vi "FileOpenWindow.vi"(8 "error in (no error)":errorcluster, 10 "Path In":string, 11 "Connection ID":T1) -> (0 "error out":errorcluster, 2 "Path Out":string, 3 "Connection ID Out":T1)   [LabVIEW 2017, in "GL860_Driver.lvlib"]
uses:
  GL860_Driver.lvlib
  Driver/ConnectionID.ctl
  <vilib>/Utility/miscctls.llb/LVPointTypeDef.ctl
panel:
  in  "Save File_Info":i32[](listbox) caption="Save File"
  in  "OK":bool
  in  "Scrollbar":i32(c297)
  out "Img 7":picture
  out "Img 6":picture
  out "Img 5":picture
  out "Img 4":picture
  out "Img 3":picture
  out "Img 2":picture
  out "Img 0":picture
  out "Img 1":picture
  out "Save File_Name":i32[](listbox) caption="Save File"
  in  "Tag":string
  in  "Pic.Temp":picture[](array[picture])=[bytes[7070], bytes[7070]]
  out "Icon":picture[](array[picture])
  out "DriveList":string[](array[string])
  out "File":string[](array[string])
  out "Folder":string[](array[string])
  in  "Device":i32(ring) items=["SD1"=-1, "-"=-2, "SD1"=0, "SD2"=1]
  in  "キャンセル":bool
  in  "Transfar":bool
  in  "Tree":string(tree)
  out "FilePath":string
  in  "Sort":u16(ring) items=["ファイル名", "更新日時"]
  in  "Send 3":bool
  in  "Send 4":bool
  # "ソート"
  # "デバイス"
  # "ファイルパス"
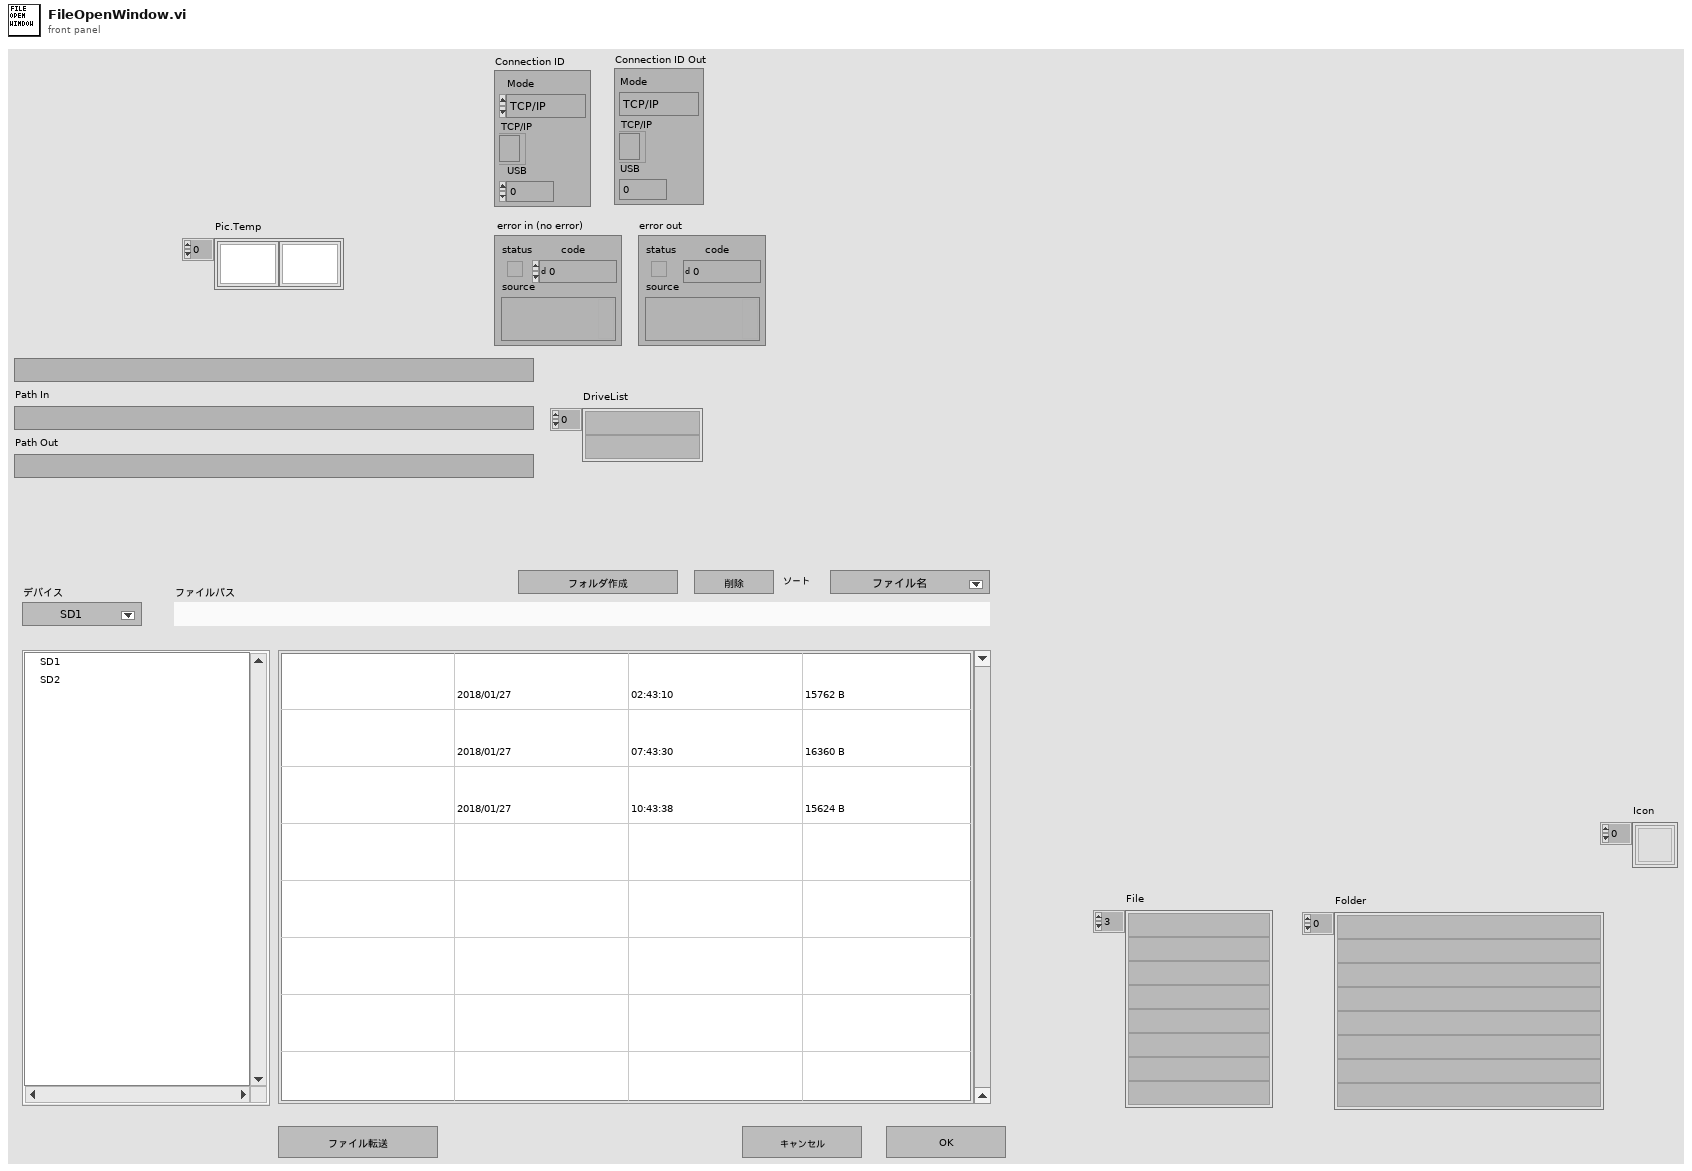
[diagram p1: front panel]
types:
  T1 = typedef "ConnectionID.ctl" = cluster{"Mode":enum16{"TCP/IP", "USB"}, "TCP/IP":refnum<k5>, "USB":i32}
  T2 = typedef "LVPointTypeDef.ctl" = cluster{"Horizontal":i16, "Vertical":i16}
  T3 = typedef "LVRowAndColumnUnsignedTypeDef.ctl" = cluster{"Row":u32, "Column":u32}
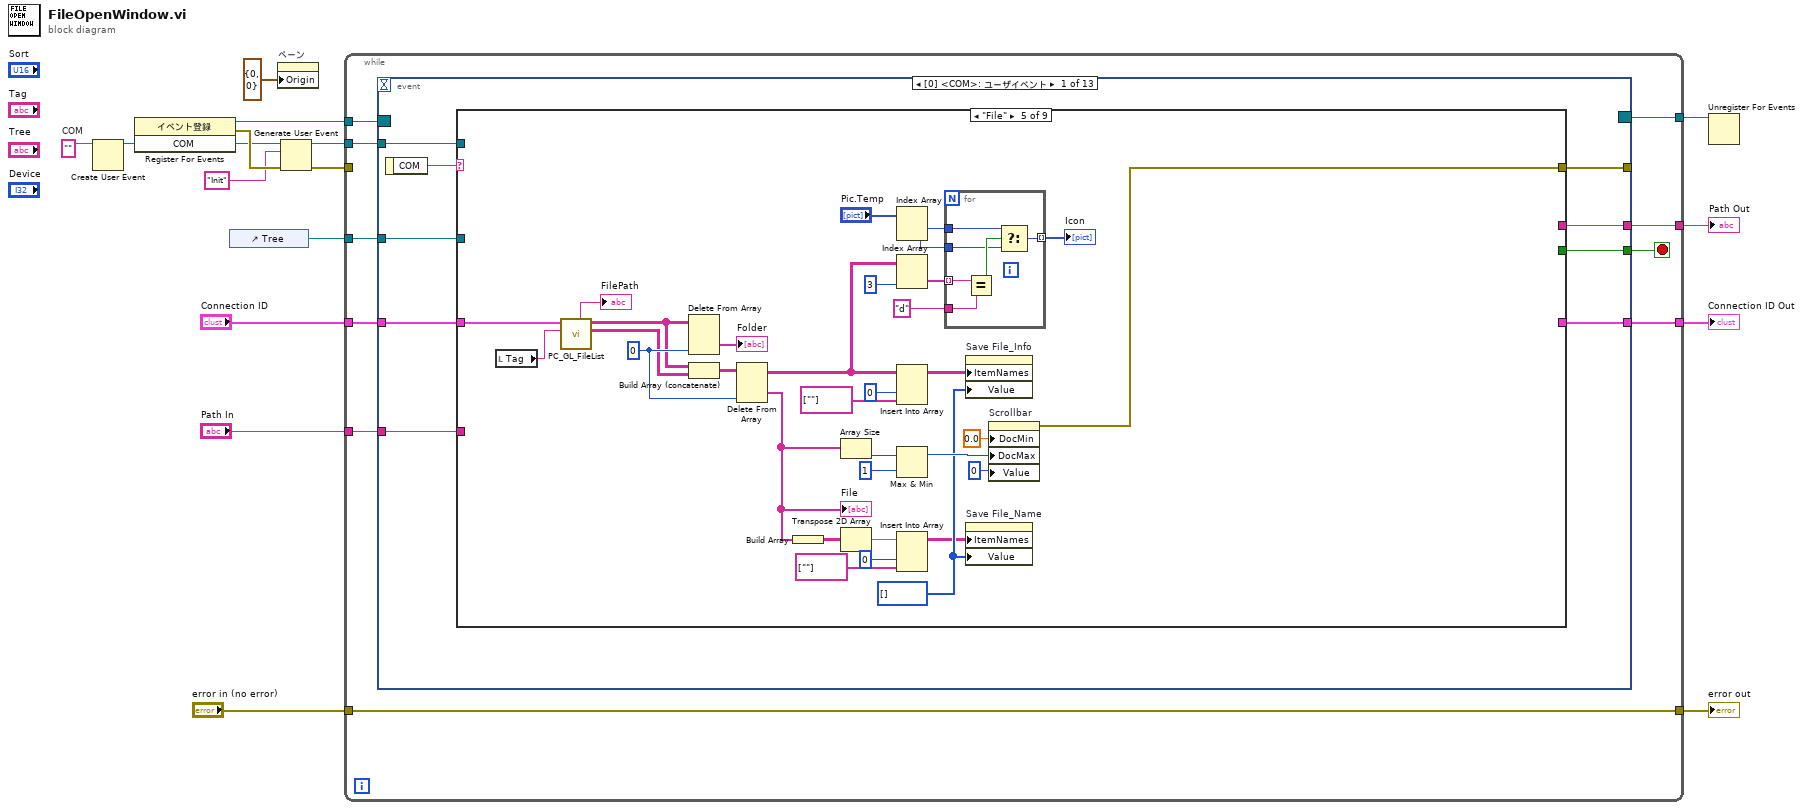
[diagram p0: block diagram]
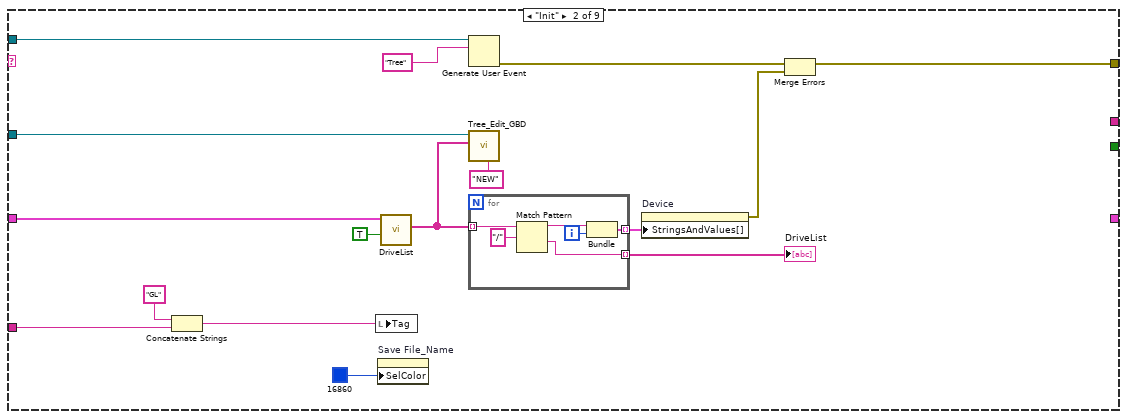
[diagram p3: hidden frame]
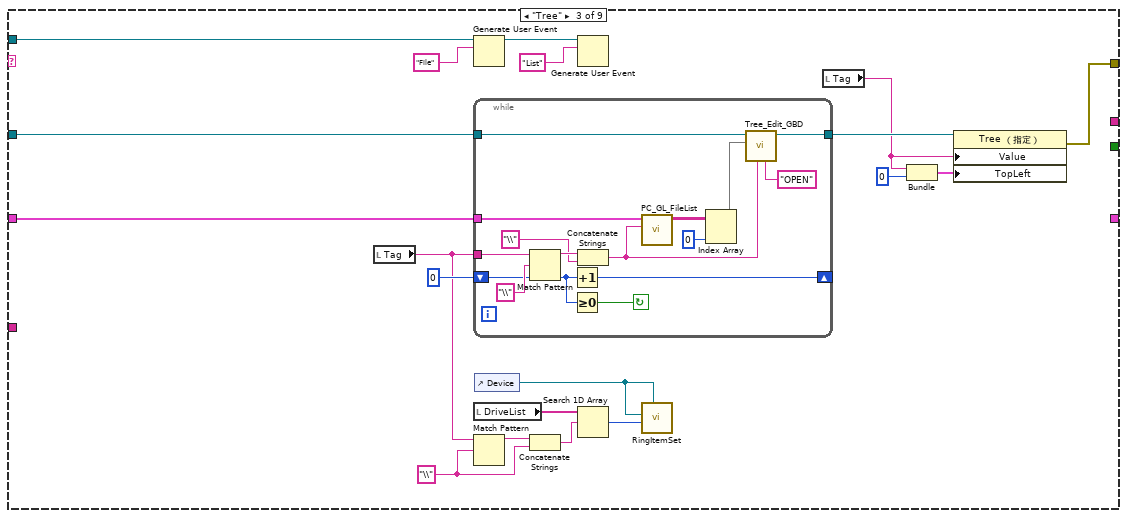
[diagram p4: hidden frame]
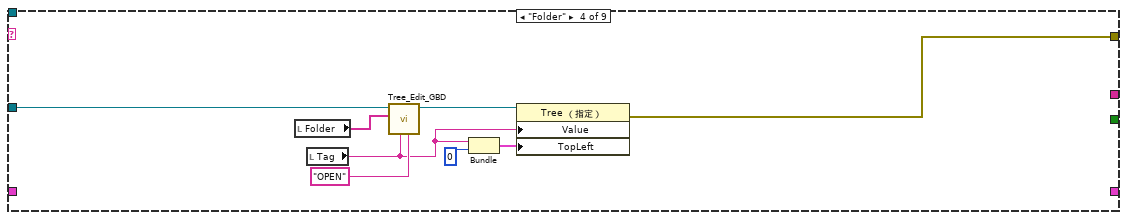
[diagram p5: hidden frame]
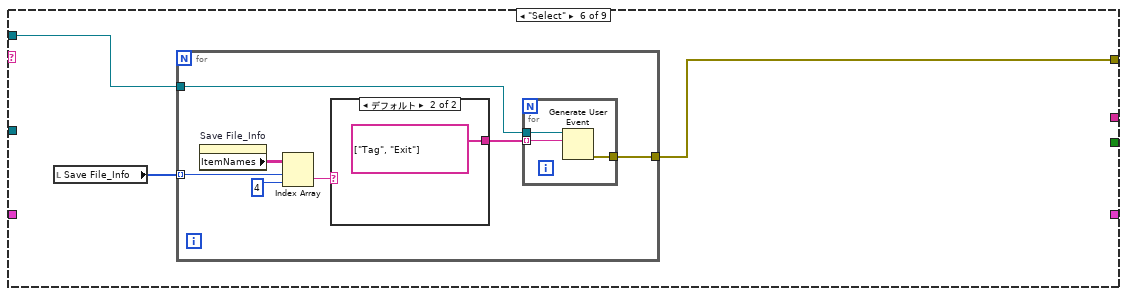
[diagram p6: hidden frame]
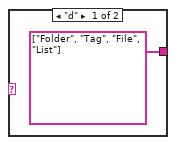
[diagram p7: hidden frame]
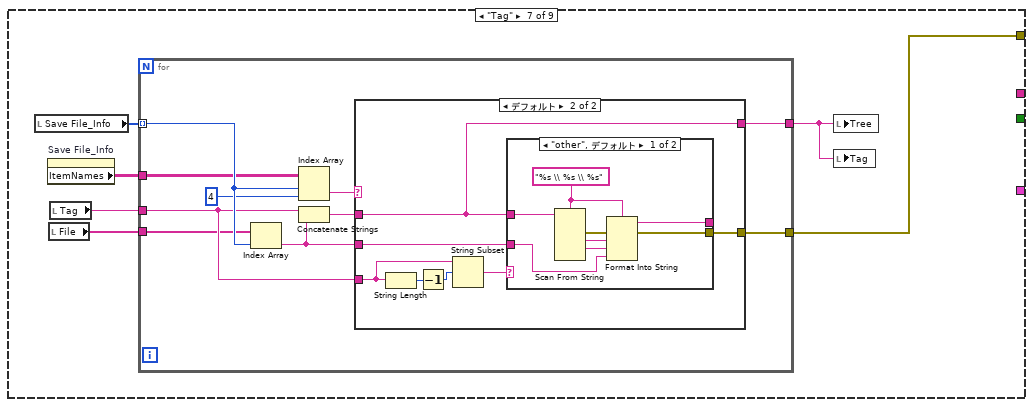
[diagram p8: hidden frame]
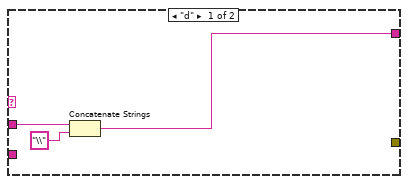
[diagram p9: hidden frame]
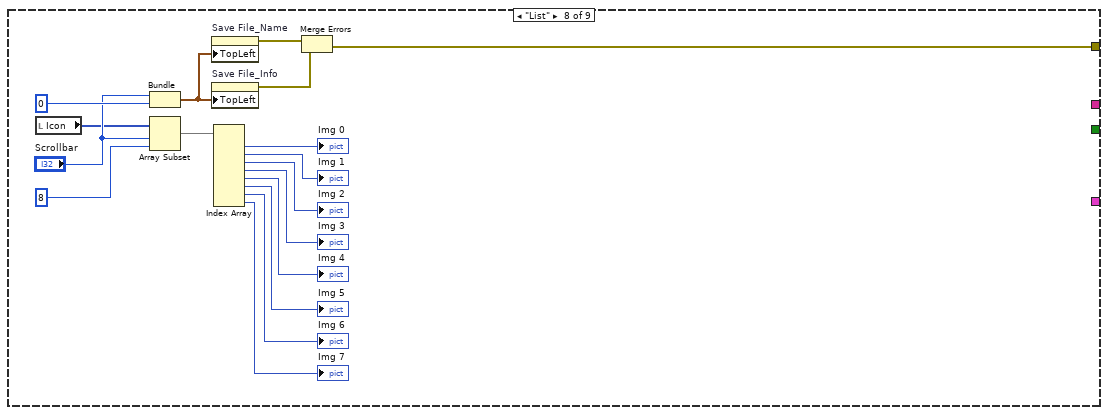
[diagram p11: hidden frame]
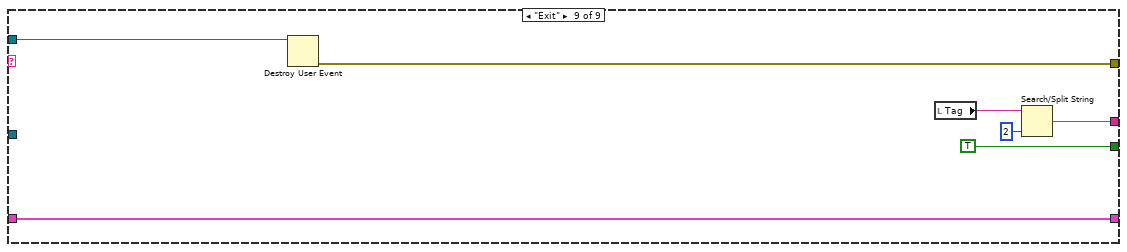
[diagram p12: hidden frame]
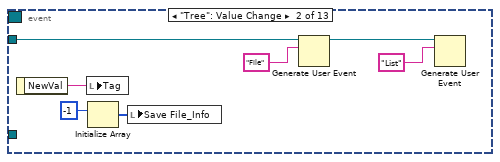
[diagram p13: hidden frame]
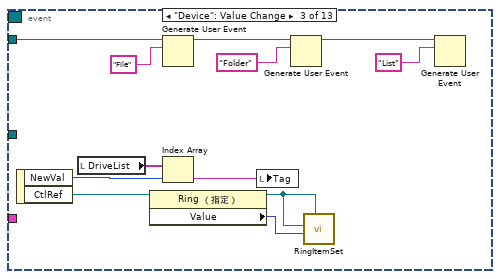
[diagram p14: hidden frame]
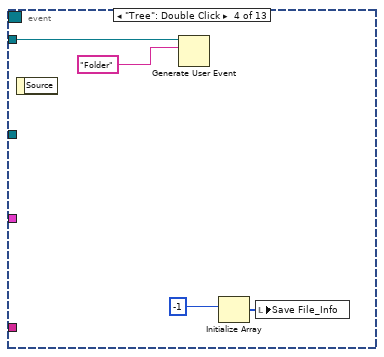
[diagram p15: hidden frame]
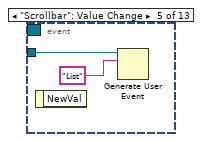
[diagram p16: hidden frame]
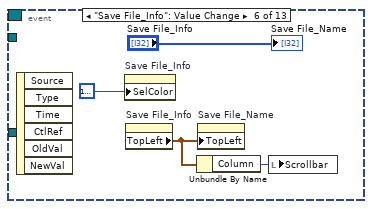
[diagram p17: hidden frame]
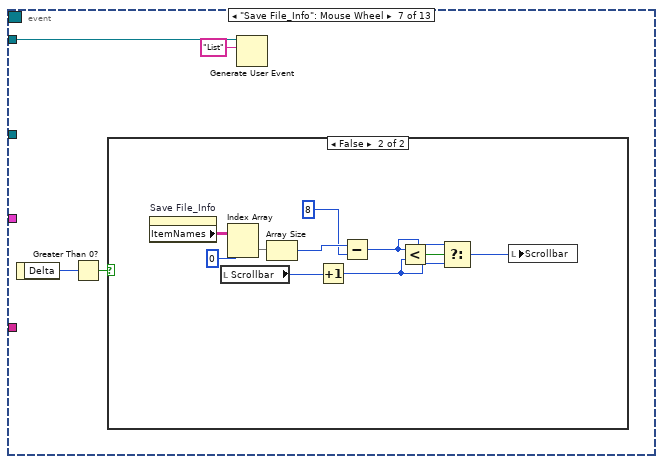
[diagram p18: hidden frame]
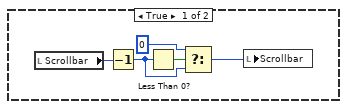
[diagram p19: hidden frame]
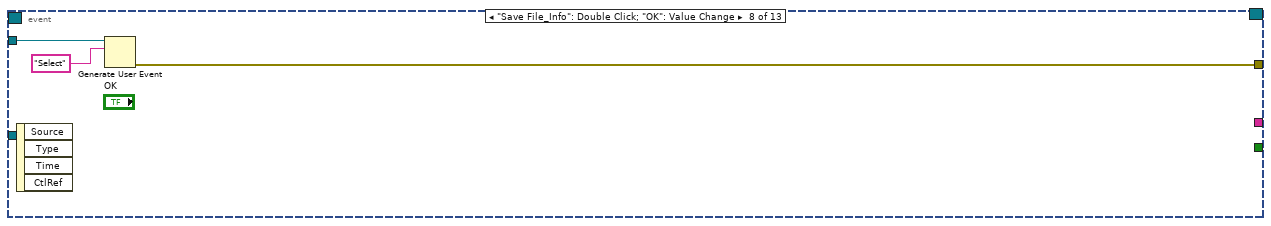
[diagram p20: hidden frame]
diagram:
  w12 = ""  # COM
  n1 = Create User Event(user event datatype=w12) -> (user event=w14:refnum<user-event>)  [unwired: 1 in, 1 out]
  n2 = register-events(w14) -> (reference out=w16:refnum<event-registration>, error out=w15:errorcluster)  [unwired: 2 in]
  n3 = control-ref of="Tree"() -> (w9:refnum<vi>)
  n4 = property on="ペーン" class="Pane"("Origin"=T2 {"Horizontal"=0, "Vertical"=0}) -> ()  [unwired: 2 in, 2 out]
  n5 = Generate User Event(user event=w14, event data cluster="Init", error in=w15) -> (user event out=w13:refnum<user-event>, error out=w3:errorcluster)  [unwired: 1 in]
  n6 = while {
    tunnel: w16 -> [w26]
    tunnel: w13 -> [w17]
    tunnel: [w24] -> w11
    tunnel: w9 -> [w23]
    tunnel: [w22] -> w8
    tunnel: "Path In" -> [w21]
    tunnel: "Connection ID" -> [w20]
    tunnel: "error in (no error)" -> [w19]
    tunnel: [w18] -> w5
    tunnel: [w19] -> w4
    tunnel: w3 -> [_]
    stop <- w25 stop-if-true
    n7 = event shown="[0] <COM>: ユーザイベント" {
      selector: w26 -> [_ _ _ _ _ _ _ _ _ _ _ _ _]
      dyn-events: [_ _ _ _ _ _ _ _ _ _ _ _ _] -> w24
      timeout: _ -> [_ _ _ _ _ _ _ _ _ _ _ _ _]
      tunnel: [w33 _ _ _ _ _ _ _ _ _ _ _ _] -> w25
      tunnel: w23 -> [w32 _ _ _ _ _ _ _ _ _ w310 _ w397]
      tunnel: [w31 _ _ _ _ _ _ _ _ _ _ _ _] -> w22
      tunnel: w21 -> [w30 _ _ _ _ _ _ _ _ _ _ _ _]
      tunnel: w20 -> [w29 _ _ _ _ _ _ _ w265 w276 w314 w370 w401]
      tunnel: [w28 _ _ _ _ _ _ _ w265 _ w313 _ w400] -> w18
      tunnel: w17 -> [w34 w217 w228 w235 w237 _ w244 w263 w268 _ w311 w341 w398]
      tunnel: [w27 _ _ _ _ _ _ w262 _ _ _ w354 _] -> _
      event User Event {
        n8 = event-data() -> ("COM"=w35:string)  [unwired: 1 in]
        n9 = case shown="\"File\"" w35 {
          tunnel: w34 -> [_ w50 w76 _ _ w142 _ _ w213]
          tunnel: [_ _ _ _ _ _ _ _ TRUE] -> w33
          tunnel: w32 -> [_ w52 w72 w100 _ _ _ _ _]
          tunnel: [_ _ _ _ _ _ _ _ w207] -> w31
          tunnel: w30 -> [_ w39 _ _ _ _ _ _ _]
          tunnel: w29 -> [w36 w48 w71 _ w133 _ _ _ w212]
          tunnel: [w36 _ _ _ _ _ _ _ w212] -> w28
          tunnel: [_ w43 w59 w95 w107 w141 w159 w191 w211] -> w27
          frame Default {
          }
          frame "Init" {
            n10 = Concatenate Strings("GL" ("string"), w39) -> (w38:string)
            n11 = local write "Tag"(w38) -> ()
            n12 = property on="Save File_Name" class="MCListbox （指定）"("SelColor"=u32 16860) -> ()  [unwired: 2 in, 2 out]
            n13 = call "DriveList.vi"("GL"=TRUE, "Connection ID"=w48) -> ("Drive"=w47:string[])  [unwired: 8 in, 1 out]
            n14 = Generate User Event(user event=w50, event data cluster="Tree") -> (error out=w42:errorcluster)  [unwired: 2 in, 1 out]
            n15 = call "Tree_Edit_GBD.vi"("MODE"="NEW", "Folder"=w47, "Tree"=w52) -> ()  [unwired: 8 in, 1 out]
            n16 = for {
              tunnel: w47 -> [w58] mode=indexing
              tunnel: [w54] -> w46 mode=indexing
              tunnel: [w55] -> w45 mode=indexing
              i -> [w53]
              n17 = Match Pattern(string=w58, regular expression="/" ("search string/char (-)")) -> (before substring=w57:string, after substring=w55:string)  [unwired: 1 in, 2 out]
              n18 = Bundle("String"=w57, w53) -> (w54:cluster{"String":string, i32})  [unwired: 1 in]
            }
            "DriveList" <- w45
            n19 = property on="Device" class="Ring （指定）"("StringsAndValues[]"=w46) -> (error out=w44:errorcluster)  [unwired: 2 in, 1 out]
            n20 = Merge Errors(w42, w44) -> (w43:errorcluster)
          }
          frame "Tree" {
            w66 = "\\" ("regular expression")
            n21 = local read "Tag"() -> (w61:string)
            n22 = Generate User Event(user event=w76, event data cluster="File") -> (user event out=w74:refnum<user-event>)  [unwired: 2 in, 1 out]
            n23 = while {
              tunnel: w72 -> [w93]
              tunnel: w61 -> [w92]
              shift-right: [w89] -> _
              shift-left: 0 ("offset past match") -> [w90]
              tunnel: w71 -> [w79]
              tunnel: [w78] -> w68
              stop <- w86 continue-if-true
              n24 = Match Pattern(string=w92, regular expression="\\", offset (0)=w90) -> (before substring=w88:string, offset past match=w87:i32)  [unwired: 2 out]
              n25 = Increment(x=w87) -> (x+1=w89:i32)
              n26 = Greater Or Equal To 0?(x=w87) -> (x >= 0?=w86:bool)
              n27 = Concatenate Strings(w88, "\\" ("regular expression")) -> (w84:string)
              n28 = call "PC_GL_FileList.vi"("Path In"=w84, "Connection ID"=w79) -> ("Folder"=w83:string[][])  [unwired: 7 in, 2 out]
              n29 = Index Array(array=w83, index (col)=0 ("disabled index (col)")) -> (element=w82:string[])  [unwired: 1 in]
              n30 = call "Tree_Edit_GBD.vi"("MODE"="OPEN", "TAG"=w84, "Folder"=w82, "Tree"=w93) -> ("Tree.Ref"=w78:refnum<vi>)  [unwired: 7 in]
            }
            n31 = local read "DriveList"() -> (w65:string[])
            n32 = Match Pattern(string=w61, regular expression=w66) -> (before substring=w67:string)  [unwired: 1 in, 3 out]
            n33 = control-ref of="Device"() -> (w63:refnum<vi>)
            n34 = Concatenate Strings(w67, w66) -> (w64:string)
            n35 = Generate User Event(user event=w74, event data cluster="List") -> ()  [unwired: 2 in, 2 out]
            n36 = Search 1D Array(1D array=w65, element=w64) -> (index of element=w62:i32)  [unwired: 1 in]
            n37 = call "RingItemSet.vi"("Target"=w63, "Value"=w62, "Base"=w63) -> ()  [unwired: 9 in]
            n38 = local read "Tag"() -> (w60:string)
            n39 = Bundle("Tag"=w60, 0) -> (w70:cluster{"Tag":string, i32})  [unwired: 1 in]
            n40 = property class="Tree （指定）"(reference=w68, "Value"=w60, "TopLeft"=w70) -> (error out=w59:errorcluster)  [unwired: 1 in, 1 out]
          }
          frame "Folder" {
            n41 = local read "Folder"() -> (w99:string[])
            n42 = local read "Tag"() -> (w94:string)
            n43 = call "Tree_Edit_GBD.vi"("MODE"="OPEN", "TAG"=w94, "Folder"=w99, "Tree"=w100) -> ("Tree.Ref"=w96:refnum<vi>)  [unwired: 7 in]
            n44 = Bundle("Tag"=w94, 0) -> (w98:cluster{"Tag":string, i32})  [unwired: 1 in]
            n45 = property class="Tree （指定）"(reference=w96, "Value"=w94, "TopLeft"=w98) -> (error out=w95:errorcluster)  [unwired: 1 in, 1 out]
          }
          frame "File" {
            w108 = i32[] [] ("Save File_Name")
            w128 = 0 ("disabled index (col)")
            n46 = local read "Tag"() -> (w111:string)
            n47 = call "PC_GL_FileList.vi"("Path In"=w111, "Connection ID"=w133) -> ("File"=w120:string[][], "Folder"=w121:string[][], "root"=→"FilePath":string)  [unwired: 7 in]
            n48 = Delete From Array(array=w121, index (col)=w128) -> (deleted portion=→"Folder":string[])  [unwired: 2 in, 1 out]
            n49 = Build Array (concatenate)(w121, w120) -> (w124:string[][])
            n50 = Delete From Array(array=w124, index (col)=w128) -> (deleted portion=w109:string[], array with subset deleted=w119:string[][])  [unwired: 2 in]
            "File" <- w109
            n51 = Build Array(w109) -> (w104:string[][])
            n52 = Array Size(array=w109) -> (size(s)=w132:i32)
            n53 = Transpose 2D Array(2D array=w104) -> (transposed array=w102:string[][])
            n54 = Index Array(array="Pic.Temp") -> (element #1=w114:picture, element #2=w113:picture)  [unwired: 2 in]
            n55 = Index Array(array=w119, index (col)=3 ("disabled index (col)")) -> (element=w118:string[])  [unwired: 1 in]
            n56 = Insert Into Array(array=w119, index (col)=0 ("disabled index (col)"), new element=string[] [""] ("new element/subarray")) -> (w110:string[][])  [unwired: 1 in]
            n57 = Max & Min(x=w132, y=1) -> (max(x,y)=w129:i32)  [unwired: 1 out]
            n58 = Insert Into Array(array=w102, index (col)=0 ("disabled index (col)"), new element=string[] [""] ("new element/subarray")) -> (w103:string[][])  [unwired: 1 in]
            n59 = for {
              tunnel: w118 -> [w139] mode=indexing
              tunnel: "d" ("Select") -> [w138]
              tunnel: w114 -> [w136]
              tunnel: w113 -> [w135]
              tunnel: [w134] -> w112 mode=indexing
              n60 = Equal?(x=w139, y=w138) -> (x = y?=w137:bool)
              n61 = Select(t=w136, s=w137, f=w135) -> (s? t:f=w134:picture)
            }
            "Icon" <- w112
            n62 = property on="Save File_Info" class="MCListbox （指定）"("ItemNames"=w110, "Value"=w108) -> ()  [unwired: 2 in, 2 out]
            n63 = property on="Save File_Name" class="MCListbox （指定）"("ItemNames"=w103, "Value"=w108) -> ()  [unwired: 2 in, 2 out]
            n64 = property on="Scrollbar" class="Scroll （指定）"("DocMin"=0.0 ("Doc Min"), "DocMax"=w129, "Value"=0 ("Scrollbar")) -> (error out=w107:errorcluster)  [unwired: 2 in, 1 out]
          }
          frame "Select" {
            n65 = local read "Save File_Info"() -> (w140:i32[])
            n66 = for {
              tunnel: w140 -> [w148] mode=indexing
              tunnel: w142 -> [w146]
              tunnel: [w143] -> w141
              n67 = property on="Save File_Info" class="MCListbox （指定）"() -> ("ItemNames"=w149:string[][])  [unwired: 2 in, 2 out]
              n68 = Index Array(array=w149, index (row)=w148, index (col)=4 ("disabled index (col)")) -> (element=w144:string)
              n69 = case shown="デフォルト" w144 {
                tunnel: [string[] ["Folder", "Tag", "File", "List"] string[] ["Tag", "Exit"]] -> w145
                frame "d" {
                }
                frame Default {
                }
              }
              n70 = for {
                tunnel: w146 -> [w152]
                tunnel: w145 -> [w151] mode=indexing
                tunnel: [w150] -> w143
                n71 = Generate User Event(user event=w152, event data cluster=w151) -> (error out=w150:errorcluster)  [unwired: 2 in, 1 out]
              }
            }
          }
          frame "Tag" {
            n72 = local read "Save File_Info"() -> (w160:i32[])
            n73 = property on="Save File_Info" class="MCListbox （指定）"() -> ("ItemNames"=w157:string[][])  [unwired: 2 in, 2 out]
            n74 = local read "File"() -> (w155:string[])
            n75 = local read "Tag"() -> (w156:string)
            n76 = for {
              tunnel: w160 -> [w170] mode=indexing
              tunnel: [w165] -> w158
              tunnel: [w164] -> w159
              tunnel: w157 -> [w163]
              tunnel: w156 -> [w162]
              tunnel: w155 -> [w161]
              n77 = Index Array(array=w161, index=w170) -> (element=w166:string)
              n78 = Index Array(array=w163, index (row)=w170, index (col)=4 ("disabled index (col)")) -> (element=w168:string)
              n79 = Concatenate Strings(w162, w166) -> (w167:string)
              n80 = case shown="デフォルト" w168 {
                tunnel: w167 -> [w173 w175]
                tunnel: [w171 w175] -> w165
                tunnel: w162 -> [_ w179]
                tunnel: w166 -> [_ w176]
                tunnel: [_ w174] -> w164
                frame "d" {
                  n81 = Concatenate Strings(w173, "\\" ("string")) -> (w171:string)
                }
                frame Default {
                  n82 = String Length(string=w179) -> (length=w180:i32)
                  n83 = Decrement(x=w180) -> (x-1=w178:i32)
                  n84 = String Subset(string=w179, offset (0)=w178) -> (substring=w177:string)  [unwired: 1 in]
                  n85 = case shown="\"other\", デフォルト" w177 {
                    tunnel: w175 -> [w188 w189]
                    tunnel: [w184 w189] -> _
                    tunnel: w176 -> [w183 _]
                    tunnel: [w181 _] -> w174
                    frame "other", Default {
                      w187 = "%s \\ %s \\ %s" ("形式文字列")
                      n86 = Scan From String(format string=w187, input string=w188) -> (error out=w182:errorcluster, output 1=w186:string, output 2=w185:string)  [unwired: 6 in, 2 out]
                      n87 = Format Into String(format string=w187, error in=w182, w186, w185, w183) -> (resulting string=w184:string, error out=w181:errorcluster)  [unwired: 1 in]
                    }
                    frame "\" " {
                    }
                  }
                }
              }
            }
            n88 = local write "Tree"(w158) -> ()
            n89 = local write "Tag"(w158) -> ()
          }
          frame "List" {
            n90 = local read "Icon"() -> (w196:picture[])
            n91 = Bundle("Scrollbar"="Scrollbar", "NewVal"=0) -> (w194:cluster{"Scrollbar":i32, "NewVal":i32})  [unwired: 1 in]
            n92 = Array Subset(array=w196, index="Scrollbar", length=8) -> (w195:picture[])
            n93 = property on="Save File_Name" class="MCListbox （指定）"("TopLeft"=w194) -> (error out=w193:errorcluster)  [unwired: 2 in, 1 out]
            n94 = property on="Save File_Info" class="MCListbox （指定）"("TopLeft"=w194) -> (error out=w192:errorcluster)  [unwired: 2 in, 1 out]
            n95 = Index Array(array=w195) -> (element #1=→"Img 0":picture, element #2=→"Img 1":picture, element #3=→"Img 2":picture, element #4=→"Img 3":picture, element #5=→"Img 4":picture, element #6=→"Img 5":picture, element #7=→"Img 6":picture, element #8=→"Img 7":picture)  [unwired: 8 in]
            n96 = Merge Errors(w193, w192) -> (w191:errorcluster)
          }
          frame "Exit" {
            n97 = Destroy User Event(user event=w213) -> (error out=w211:errorcluster)  [unwired: 1 in]
            n98 = local read "Tag"() -> (w208:string)
            n99 = Search/Split String(string=w208, offset (0)=2) -> (match + rest of string=w207:string)  [unwired: 3 out]
          }
        }
      }
      event "Tree": Value Change {
        n100 = event-data() -> ("NewVal"=w214:string)  [unwired: 1 in]
        n101 = local write "Tag"(w214) -> ()
        n102 = Initialize Array(-1 ("要素")) -> (w216:i32[])  [unwired: 1 in]
        n103 = local write "Save File_Info"(w216) -> ()
        n104 = Generate User Event(user event=w217, event data cluster="File") -> (user event out=w218:refnum<user-event>)  [unwired: 2 in, 1 out]
        n105 = Generate User Event(user event=w218, event data cluster="List") -> ()  [unwired: 2 in, 2 out]
      }
      event "Device": Value Change {
        n106 = event-data() -> ("NewVal"=w232:i32, "CtlRef"=w223:refnum<vi>)  [unwired: 1 in]
        n107 = local read "DriveList"() -> (w222:string[])
        n108 = property on="Property Node" class="Ring （指定）"(reference=w223) -> (reference out=w224:refnum<vi>, "Value"=w225:i32)  [unwired: 1 in, 1 out]
        n109 = Generate User Event(user event=w228, event data cluster="File") -> (user event out=w227:refnum<user-event>)  [unwired: 2 in, 1 out]
        n110 = Index Array(array=w222, index=w232) -> (element=w221:string)
        n111 = local write "Tag"(w221) -> ()
        n112 = Generate User Event(user event=w227, event data cluster="Folder") -> (user event out=w226:refnum<user-event>)  [unwired: 2 in, 1 out]
        n113 = call "RingItemSet.vi"("Target"=w224, "Value"=w225, "Base"=w224) -> ()  [unwired: 9 in]
        n114 = Generate User Event(user event=w226, event data cluster="List") -> ()  [unwired: 2 in, 2 out]
      }
      event "Tree": Double Click {
        n115 = event-data() -> ()  [unwired: 1 in, 1 out]
        n116 = Generate User Event(user event=w235, event data cluster="Folder") -> ()  [unwired: 2 in, 2 out]
        n117 = Initialize Array(-1) -> (w233:i32[])  [unwired: 1 in]
        n118 = local write "Save File_Info"(w233) -> ()
      }
      event "Scrollbar": Value Change {
        n119 = event-data() -> ()  [unwired: 1 in, 1 out]
        n120 = Generate User Event(user event=w237, event data cluster="List") -> ()  [unwired: 2 in, 2 out]
      }
      event "Save File_Info": Value Change {
        n121 = event-data() -> ()  [unwired: 1 in, 6 out]
        n122 = property on="Save File_Info" class="MCListbox （指定）"("SelColor"=u32 16777216) -> ()  [unwired: 2 in, 2 out]
        n123 = property on="Save File_Info" class="MCListbox （指定）"() -> ("TopLeft"=w240:T3)  [unwired: 2 in, 2 out]
        n124 = Unbundle By Name(w240) -> ("Column"=w241:u32)
        n125 = property on="Save File_Name" class="MCListbox （指定）"("TopLeft"=w240) -> ()  [unwired: 2 in, 2 out]
        n126 = local write "Scrollbar"(w241) -> ()
        "Save File_Name" <- "Save File_Info"
      }
      event "Save File_Info": Mouse Wheel {
        n127 = event-data() -> ("Delta"=w246:i32)  [unwired: 1 in]
        n128 = Greater Than 0?(x=w246) -> (x > 0?=w245:bool)
        n129 = case shown="FALSE" w245 {
          frame True {
            n130 = local read "Scrollbar"() -> (w251:i32)
            n131 = Decrement(x=w251) -> (x-1=w248:i32)
            n132 = Less Than 0?(x=w248) -> (x < 0?=w250:bool)
            n133 = Select(t=0, s=w250, f=w248) -> (s? t:f=w247:i32)
            n134 = local write "Scrollbar"(w247) -> ()
          }
          frame False {
            n135 = property on="Save File_Info" class="MCListbox （指定）"() -> ("ItemNames"=w260:string[][])  [unwired: 2 in, 2 out]
            n136 = local read "Scrollbar"() -> (w261:i32)
            n137 = Index Array(array=w260, index (col)=0 ("無効な指標 （列）")) -> (element=w259:string[])  [unwired: 1 in]
            n138 = Array Size(array=w259) -> (size(s)=w257:i32)
            n139 = Increment(x=w261) -> (x+1=w256:i32)
            n140 = Subtract(x=w257, y=8) -> (x-y=w253:i32)
            n141 = Less?(x=w253, y=w256) -> (x < y?=w258:bool)
            n142 = Select(t=w253, s=w258, f=w256) -> (s? t:f=w255:i32)
            n143 = local write "Scrollbar"(w255) -> ()
          }
        }
        n144 = Generate User Event(user event=w244, event data cluster="List" ("イベントデータ")) -> ()  [unwired: 2 in, 2 out]
      }
      event "Save File_Info": Double Click; "OK": Value Change {
        n145 = event-data() -> ()  [unwired: 1 in, 4 out]
        n146 = Generate User Event(user event=w263, event data cluster="Select") -> (error out=w262:errorcluster)  [unwired: 2 in, 1 out]
      }
      event "キャンセル": Value Change {
        n147 = event-data() -> ()  [unwired: 1 in, 6 out]
        n148 = Generate User Event(user event=w268, event data cluster="Exit") -> ()  [unwired: 2 in, 2 out]
        n149 = local write "Tag"("" ("Tag")) -> ()
      }
      event "Transfar": Value Change {
        n150 = event-data() -> ()  [unwired: 1 in, 1 out]
        n151 = local read "Save File_Info"() -> (w270:i32[])
        n152 = local read "Tag"() -> (w275:string)
        n153 = local read "File"() -> (w272:string[])
        n154 = case shown="\"GLRAM\\\\\"" w275 {
          selector: w275 -> [_ w283]
          tunnel: ["GL" w283] -> w274
          tunnel: [string[] ["RAM.GBD"] ("File") w282] -> w273
          tunnel: w272 -> [_ w282]
          tunnel: [i32[] [0] ("Save File_Info") w281] -> w271
          tunnel: w270 -> [_ w281]
          tunnel: [TRUE _] -> w269
          frame "GLRAM\\" {
          }
          frame Default {
          }
        }
        n155 = for {
          tunnel: w276 -> [w294]
          tunnel: w271 -> [w292] mode=indexing
          tunnel: w273 -> [w291]
          tunnel: w274 -> [w285]
          tunnel: w269 -> [w284]
          n156 = Index Array(array=w291, index=w292) -> (element=w286:string)
          n157 = Concatenate Strings(w285, w286) -> (w290:string)
          n158 = Search/Split String(string=w290, offset (0)=2) -> (match + rest of string=w289:string)  [unwired: 1 in, 2 out]
          n159 = File Dialog(9:w286) -> (0:w293:errorcluster, 1:w296:bool, 3:w295:path)  [unwired: 6 in, 1 out]
          n160 = Concatenate Strings("\\" ("文字列"), w289) -> (w287:string)
          n161 = case shown="FALSE" w296 {
            tunnel: w294 -> [w302 _]
            tunnel: w287 -> [w301 _]
            tunnel: w295 -> [w300 _]
            tunnel: w293 -> [w299 _]
            tunnel: w284 -> [w298 _]
            frame False {
              n162 = case shown="TRUE" w298 {
                tunnel: w302 -> [w306 w309]
                tunnel: w301 -> [w305 _]
                tunnel: w300 -> [w304 w307]
                tunnel: w299 -> [w303 w308]
                frame False {
                  n163 = call "Smp_Data_transfer.vi"("Connection ID"=w306, "SaveFilePath"=w304, "Source file path"=w305, "error in (no error)"=w303) -> ()  [unwired: 7 in, 5 out]
                }
                frame True {
                  n164 = call "Smp_RAM_transfer.vi"("Connection ID"=w309, "SaveFilePath"=w307, "error in (no error)"=w308) -> ()  [unwired: 8 in, 5 out]
                }
              }
            }
            frame True {
            }
          }
        }
      }
      event "Send 4": Value Change {
        n165 = event-data() -> ()  [unwired: 1 in, 6 out]
        n166 = flat-sequence {
          tunnel: w314 -> [w319]
          tunnel: [w318] -> w312
          tunnel: w310 -> [w317]
          tunnel: [w334] -> w313
          tunnel: w312 -> [w334]
          tunnel: w311 -> [w328]
          frame #0 {
            n167 = call "CreateFolder.vi"() -> ("Bool"=w315:bool, "Return"=w316:string)  [unwired: 10 in]
            n168 = case shown="FALSE" w315 {
              tunnel: w319 -> [w326 w327]
              tunnel: [w325 w327] -> w318
              tunnel: w317 -> [w324 _]
              tunnel: w316 -> [w320 _]
              frame False {
                n169 = local read "Tag"() -> (w321:string)
                n170 = Build Array(w320) -> (w323:string[])
                n171 = call "GLdrv_FILE_MD.vi"("Connection ID"=w326, "Folder"=w320) -> ("Connection ID Out"=w325:T1)  [unwired: 1 in, 12 out]
                n172 = call "Tree_Edit_GBD.vi"("MODE"="ADD", "TAG"=w321, "Folder"=w323, "Tree"=w324) -> ()  [unwired: 7 in, 1 out]
              }
              frame True {
              }
            }
          }
          frame #1 {
            n173 = Generate User Event(user event=w328, event data cluster="Tree" ("イベントデータ")) -> (user event out=w329:refnum<user-event>)  [unwired: 2 in, 1 out]
            n174 = Generate User Event(user event=w329, event data cluster="File" ("イベントデータ")) -> (user event out=w332:refnum<user-event>)  [unwired: 2 in, 1 out]
            n175 = Generate User Event(user event=w332, event data cluster="List") -> ()  [unwired: 2 in, 2 out]
          }
        }
      }
      event "Sort": Value Change {
        w335 = i32[] [] ("Save File_Name")
        n176 = event-data() -> ("NewVal"=w362:u16)  [unwired: 1 in, 5 out]
        n177 = local read "Tag"() -> (w369:string)
        n178 = call "PC_GL_FileList.vi"("Path In"=w369, "Connection ID"=w370) -> ("File"=w367:string[][], "Folder"=w368:string[][])  [unwired: 7 in, 1 out]
        n179 = Generate User Event(user event=w341, event data cluster="List") -> ()  [unwired: 2 in, 2 out]
        n180 = Build Array (concatenate)(w368, w367) -> (w364:string[][])
        n181 = case shown="1" w362 {
          tunnel: w364 -> [w385 w392]
          tunnel: [w385 w387] -> w363
          frame 0, Default {
          }
          frame 1 {
            n182 = Delete From Array(array=w392, length=2 ("長さ"), index (col)=1 ("指標 （行）")) -> (deleted portion=w388:string[][], array with subset deleted=w389:string[][])  [unwired: 1 in]
            n183 = Insert Into Array(array=w389, index (col)=0 ("無効な指標 （列）"), new element=w388) -> (w387:string[][])  [unwired: 1 in]
          }
        }
        n184 = for {
          tunnel: w363 -> [w396] mode=indexing
          tunnel: [w395] -> w366 mode=indexing
          n185 = Bundle(w396) -> (w395:cluster{string[]})  [unwired: 1 in]
        }
        n186 = Sort 1D Array(array=w366) -> (sorted array=w365:cluster{string[]}[])
        n187 = for {
          tunnel: w365 -> [w394] mode=indexing
          tunnel: [w393] -> w361 mode=indexing
          n188 = Unbundle(w394) -> (w393:string[])
        }
        n189 = case shown="1" w362 {
          tunnel: w361 -> [w377 w384]
          tunnel: [w377 w380] -> w344
          frame 0, Default {
          }
          frame 1 {
            n190 = Delete From Array(array=w384, length=2 ("長さ"), index (col)=0 ("指標 （行）")) -> (deleted portion=w381:string[][], array with subset deleted=w382:string[][])  [unwired: 1 in]
            n191 = Insert Into Array(array=w382, index (col)=1 ("指標 （行）"), new element=w381) -> (w380:string[][])  [unwired: 1 in]
          }
        }
        n192 = local read "Pic.Temp"() -> (w346:picture[])
        n193 = Delete From Array(array=w344, index (col)=0 ("無効な指標 （列）")) -> (deleted portion=w338:string[], array with subset deleted=w343:string[][])  [unwired: 2 in]
        n194 = Array Size(array=w338) -> (size(s)=w355:i32)
        n195 = Index Array(array=w346) -> (element #1=w348:picture, element #2=w347:picture)  [unwired: 2 in]
        n196 = Index Array(array=w343, index (col)=3 ("disabled index (col)")) -> (element=w351:string[])  [unwired: 1 in]
        n197 = Max & Min(x=w355, y=1) -> (max(x,y)=w358:i32)  [unwired: 1 out]
        n198 = Build Array(string[] [""] ("new element/subarray"), w338) -> (w337:string[][])
        n199 = for {
          tunnel: w351 -> [w376] mode=indexing
          tunnel: "d" ("Select") -> [w375]
          tunnel: w348 -> [w373]
          tunnel: w347 -> [w372]
          tunnel: [w371] -> w345 mode=indexing
          n200 = Equal?(x=w376, y=w375) -> (x = y?=w374:bool)
          n201 = Select(t=w373, s=w374, f=w372) -> (s? t:f=w371:picture)
        }
        n202 = property on="Scrollbar" class="Scroll （指定）"("DocMin"=0.0 ("Doc Min"), "DocMax"=w358, "Value"=0 ("Scrollbar")) -> (error out=w354:errorcluster)  [unwired: 2 in, 1 out]
        n203 = Insert Into Array(array=w343, index (col)=0 ("disabled index (col)"), new element=string[] [""] ("new element/subarray")) -> (w340:string[][])  [unwired: 1 in]
        n204 = Transpose 2D Array(2D array=w337) -> (transposed array=w336:string[][])
        n205 = property on="Save File_Info" class="MCListbox （指定）"("ItemNames"=w340, "Value"=w335) -> ()  [unwired: 2 in, 2 out]
        n206 = property on="Save File_Name" class="MCListbox （指定）"("ItemNames"=w336, "Value"=w335) -> ()  [unwired: 2 in, 2 out]
        n207 = local write "Icon"(w345) -> ()
      }
      event "Send 3": Value Change {
        n208 = event-data() -> ()  [unwired: 1 in, 6 out]
        n209 = flat-sequence {
          tunnel: w401 -> [w407]
          tunnel: [w406] -> w399
          tunnel: w397 -> [w405]
          tunnel: [w451] -> w400
          tunnel: w399 -> [w451]
          tunnel: w398 -> [w447]
          frame #0 {
            n210 = local read "File"() -> (w404:string[])
            n211 = local read "Tag"() -> (w403:string)
            n212 = property on="Save File_Info" class="MCListbox （指定）"() -> ("ItemNames"=w402:string[][])  [unwired: 2 in, 2 out]
            n213 = local read "Save File_Info"() -> (w408:i32[])
            n214 = for {
              tunnel: w408 -> [w413] mode=indexing
              tunnel: w407 -> [w421]
              tunnel: [w420] -> w406
              tunnel: w405 -> [w414]
              tunnel: w404 -> [w412]
              tunnel: w403 -> [w409]
              tunnel: w402 -> [w411]
              n215 = Index Array(array=w412, index=w413) -> (element=w410:string)
              n216 = Concatenate Strings(w409, w410) -> (w419:string)
              n217 = Index Array(array=w411, index (row)=w413, index (col)=4 ("disabled index (col)")) -> (element=w422:string)
              n218 = String Subset(string=w419, offset (0)=2 ("オフセット（0）")) -> (substring=w416:string)  [unwired: 1 in]
              n219 = Concatenate Strings("\\" ("文字列"), w416) -> (w417:string)
              n220 = case shown="\"d\"" w422 {
                tunnel: w417 -> [w434 w439]
                tunnel: w421 -> [w430 w442]
                tunnel: [w429 w441] -> w420
                tunnel: w414 -> [w431 w438]
                tunnel: w410 -> [w427 w436]
                tunnel: w409 -> [w424 w435]
                frame "d" {
                  n221 = Concatenate Strings(w434, "\\" ("文字列")) -> (w428:string)
                  n222 = call "Alldelete.vi"("Connection ID Out"=w430, "Strings"=w428) -> ("Connection ID"=w429:T1)  [unwired: 12 in, 1 out]
                  n223 = Concatenate Strings(w424, w427, "\\" ("文字列")) -> (w426:string)
                  n224 = call "Tree_Edit_GBD.vi"("MODE"="DEL", "TAG"=w426, "Tree"=w431) -> ()  [unwired: 8 in, 1 out]
                }
                frame Default {
                  n225 = call "GLdrv_FILE_RM.vi"("Connection ID"=w442, "File Path"=w439) -> ("Connection ID Out"=w441:T1)  [unwired: 1 in, 12 out]
                  n226 = Concatenate Strings(w435, w436) -> (w437:string)
                  n227 = call "Tree_Edit_GBD.vi"("MODE"="DEL", "TAG"=w437, "Tree"=w438) -> ()  [unwired: 8 in, 1 out]
                }
              }
            }
          }
          frame #1 {
            n228 = Generate User Event(user event=w447, event data cluster="File" ("イベントデータ")) -> (user event out=w449:refnum<user-event>)  [unwired: 2 in, 1 out]
            n229 = Initialize Array(-1 ("要素")) -> (w444:i32[])  [unwired: 1 in]
            n230 = local write "Save File_Info"(w444) -> ()
            n231 = Generate User Event(user event=w449, event data cluster="List") -> (user event out=w445:refnum<user-event>)  [unwired: 2 in, 1 out]
            n232 = Generate User Event(user event=w445, event data cluster="Tree") -> ()  [unwired: 2 in, 2 out]
          }
        }
      }
    }
  }
  "Path Out" <- w8
  "error out" <- w4
  "Connection ID Out" <- w5
  n233 = Unregister For Events(event registration refnum=w11) -> ()  [unwired: 1 in, 1 out]
